vi "Write Active Item Tag.vi"(8 "error in (no error)":errorcluster, 10 "ActiveItemTag":string, 11 "TreeControl.lvclass in":refnum<class "TreeControl.lvclass">) -> (0 "error out":errorcluster, 3 "TreeControl.lvclass out":refnum<class "TreeControl.lvclass">)   [LabVIEW 2015, in "TreeControl.lvclass"]
uses:
  TreeControl.lvclass
  TreeControl.lvclass/TreeControl.ctl
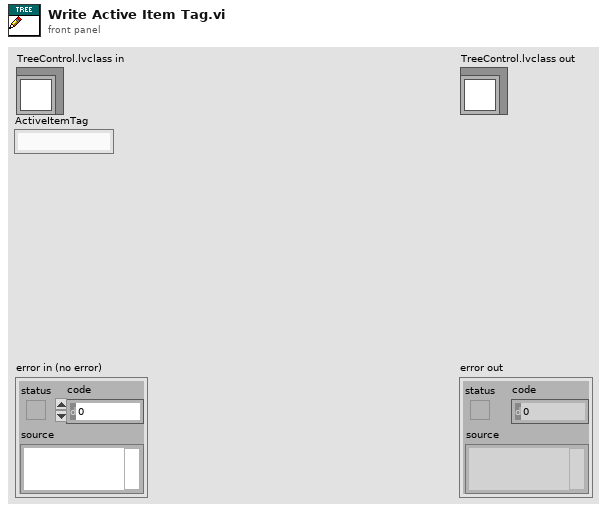
[diagram p1: front panel]
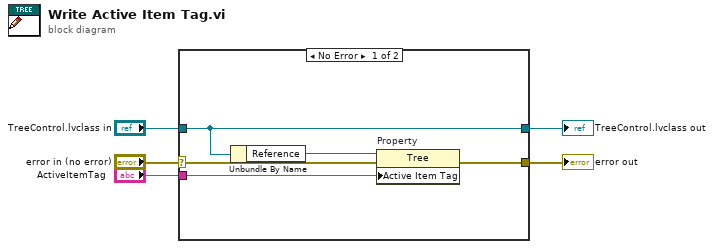
[diagram p0: block diagram]
diagram:
  n1 = case shown="No Error" "error in (no error)" {
    selector: "error in (no error)" -> [w6 w12]
    tunnel: [w10 w12] -> w4
    tunnel: [w8 w11] -> w2
    tunnel: "TreeControl.lvclass in" -> [w8 w11]
    tunnel: "ActiveItemTag" -> [w9 _]
    frame No Error {
      n2 = Unbundle By Name(w8) -> ("Reference"=w7:refnum<vi>)
      n3 = property on="Property" class="Tree"(reference=w7, error in=w6, "Active Item Tag"=w9) -> (error out=w10:errorcluster)  [unwired: 1 out]
    }
    frame Error {
    }
  }
  "error out" <- w4
  "TreeControl.lvclass out" <- w2
